vi "Set_Init.vi"(8 "error in (no error)":errorcluster, 10 "Init":bool, 11 "NKT in":refnum<class "NKT.lvclass">) -> (0 "error out":errorcluster, 3 "NKT out":refnum<class "NKT.lvclass">)   [LabVIEW 2018, in "NKT.lvclass"]
uses:
  <instrlib>/Classes/Laser/NKT/NKT.lvclass
  <instrlib>/Classes/Laser/NKT/NKT.lvclass/NKT.ctl
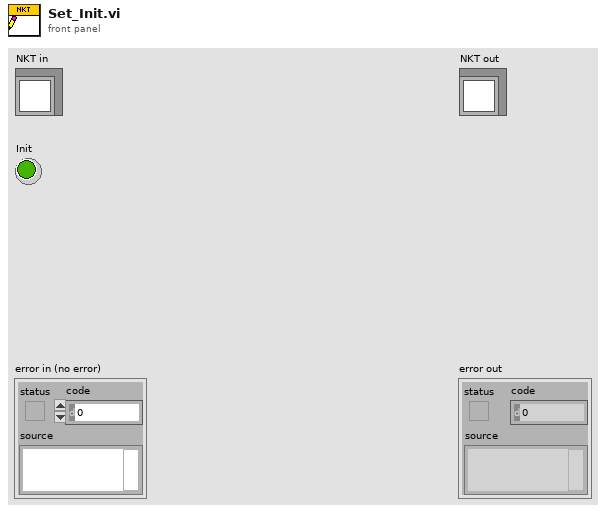
[diagram p1: front panel]
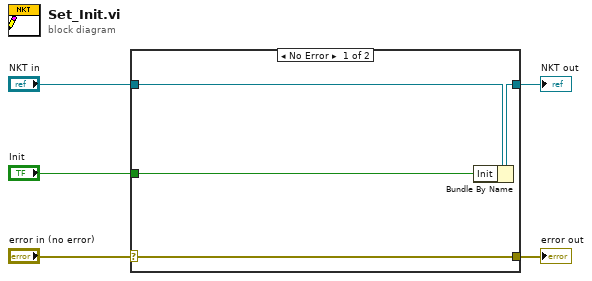
[diagram p0: block diagram]
diagram:
  n1 = case shown="No Error" "error in (no error)" {
    selector: "error in (no error)" -> [w9 w10]
    tunnel: [w9 w10] -> w4
    tunnel: [w7 w11] -> w2
    tunnel: "NKT in" -> [w8 w11]
    tunnel: "Init" -> [w6 _]
    frame No Error {
      n2 = Bundle By Name(cluster=w8, "Init"=w6) -> (w7:refnum<class "NKT.lvclass">)
    }
    frame Error {
    }
  }
  "error out" <- w4
  "NKT out" <- w2
